vi "RT Errors.New Allocated String.vi"   [LabVIEW 2016, in "RT Error Handling.lvlib"]
uses:
  RT Error Handling.lvlib
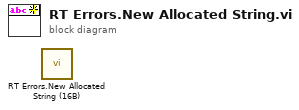
[diagram p0: block diagram]
diagram:
  n1 = call "RT Errors.New Allocated String (16B).vi"() -> ()  [unwired: 11 in, 1 out]
